vi "test-swerve-drive-kinematics-15.vi"() -> (3 "Test Passed":bool)   [LabVIEW 2019]
uses:
  <vilib>/Rock Robotics/WPI/ThirdParty/JAS_Junk/TrajLib/Conv_Deg_Radians.vi
  <vilib>/Rock Robotics/WPI/ThirdParty/JAS_Junk/TrajLib/Rotation2d_CreateAngle.vi
  <vilib>/Rock Robotics/WPI/ThirdParty/JAS_Junk/TrajLib/Trajectory_Library.lvlib
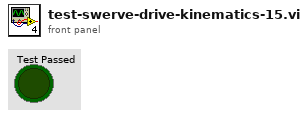
[diagram p1: front panel]
types:
  T1 = typedef "Trajectory_Library.lvlib/ROTATION2D.ctl" = cluster{"VALUE":dbl, "COS":dbl, "SIN":dbl}
  T2 = typedef "Trajectory_Library.lvlib/TRANSLATION2D.ctl" = cluster{"X":dbl, "Y":dbl}
  T3 = typedef "Trajectory_Library.lvlib/SWERVE_DRIVE_MODULE_POSITION.ctl" = cluster{"Distance":dbl, "Angle":T1}
  T4 = typedef "Trajectory_Library.lvlib/SWERVE_DRIVE_KINEMATICS.ctl" = cluster{"NumModules":i32, "InverseKinematics":T5, "ForwardKinematics":T5, "Modules":T2[], "PrevCoR":T2, "SavedModuleStates":T6[]}
  T5 = typedef "NI_Matrix.lvlib/RealMatrix.ctl" = dbl[][]
  T6 = typedef "Trajectory_Library.lvlib/SWERVE_DRIVE_MODULE_STATE.ctl" = cluster{"Speed":dbl, "Angle":T1}
  T7 = typedef "Trajectory_Library.lvlib/TWIST2D.ctl" = cluster{"dX":dbl, "dY":dbl, "dTHETA":dbl}
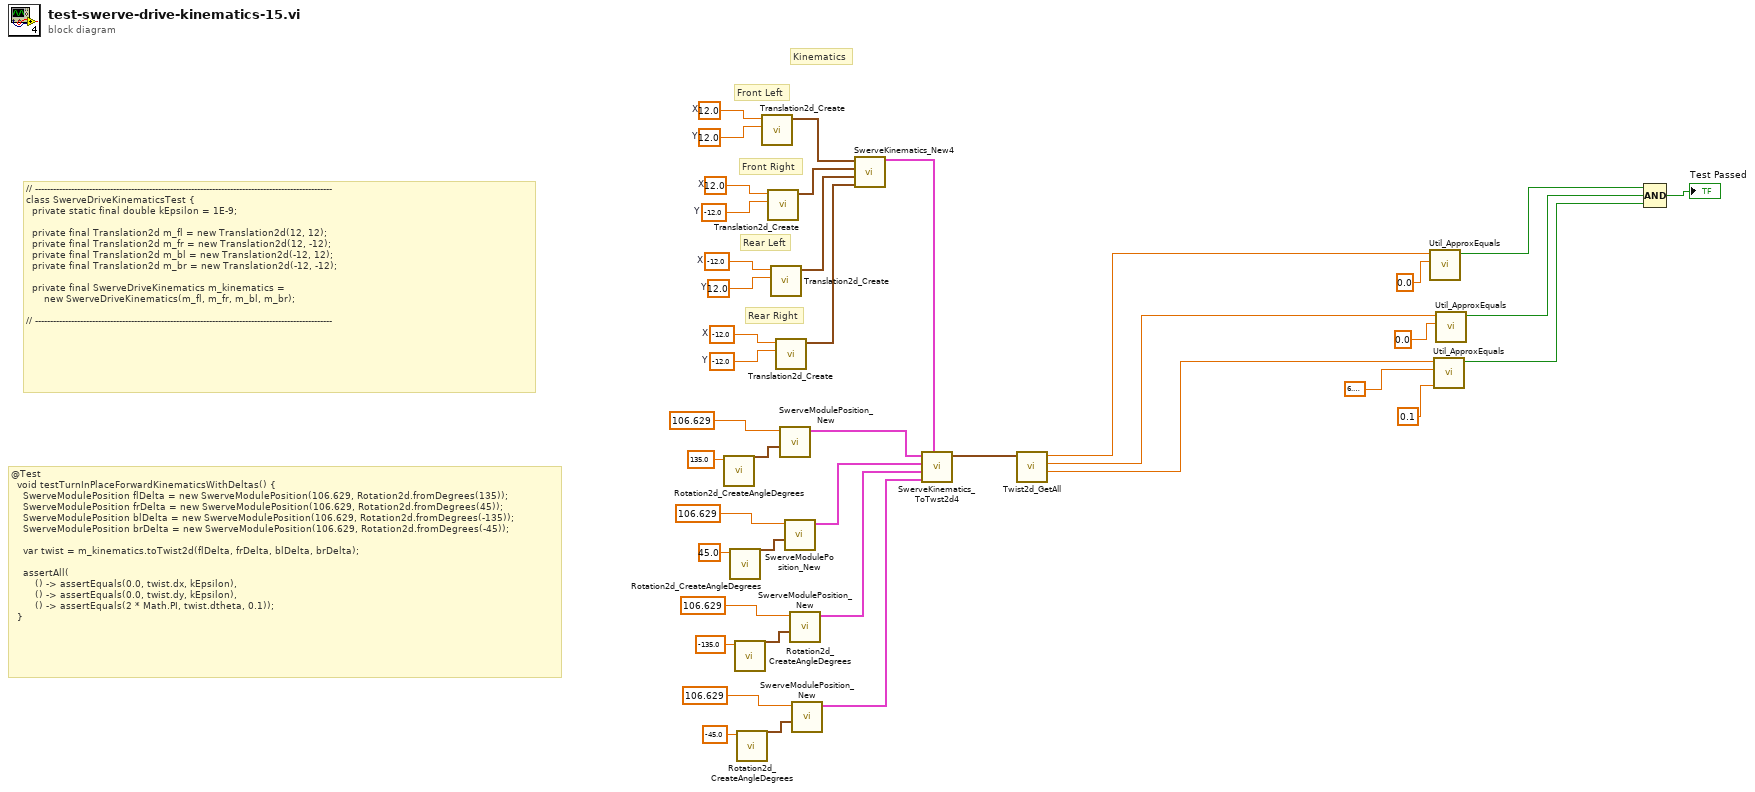
[diagram p0: block diagram]
diagram:
  w37 = -12.0  # X
  w36 = -12.0  # Y
  w35 = -12.0  # X
  w34 = 12.0  # Y
  w33 = 12.0  # X
  w32 = -12.0  # Y
  w31 = 12.0  # X
  w30 = 12.0  # Y
  # "@Test\n  void testTurnInPlaceForwardKinematicsWithDeltas() {\n    SwerveModulePosition flDelta = new SwerveModulePosition(106.629, Rotation2d.fromDegrees(135));\n    SwerveModulePosition frDelta = new SwerveModulePosition(106.629, Rotation2d.fromDegrees(45));\n    SwerveModulePosition blDelta = new SwerveModulePosition(106.629, Rotation2d.fromDegrees(-135));\n    SwerveModulePosition brDelta = new SwerveModulePosition(106.629, Rotation2d.fromDegrees(-45));\n\n    var twist = m_kinematics.toTwist2d(flDelta, frDelta, blDelta, brDelta);\n\n    assertAll(\n        () -> assertEquals(0.0, twist.dx, kEpsilon),\n        () -> assertEquals(0.0, twist.dy, kEpsilon),\n        () -> assertEquals(2 * Math.PI, twist.dtheta, 0.1));\n  }"
  # "Kinematics"
  # "Rear Right"
  # "Rear Left"
  # "Front Right"
  # "Front Left"
  # "// ---------------------------------------------------------------------------------------------------\nclass SwerveDriveKinematicsTest {\n  private static final double kEpsilon = 1E-9;\n\n  private final Translation2d m_fl = new Translation2d(12, 12);\n  private final Translation2d m_fr = new Translation2d(12, -12);\n  private final Translation2d m_bl = new Translation2d(-12, 12);\n  private final Translation2d m_br = new Translation2d(-12, -12);\n\n  private final SwerveDriveKinematics m_kinematics =\n      new SwerveDriveKinematics(m_fl, m_fr, m_bl, m_br);\n\n// ---------------------------------------------------------------------------------------------------"
  n1 = call <vilib>:"Rotation2d_CreateAngleDegrees.vi"("Angle_Degrees"=135.0) -> ("ROTATION"=w23:T1)  [unwired: 10 in]
  n2 = call <vilib>:"Rotation2d_CreateAngleDegrees.vi"("Angle_Degrees"=45.0) -> ("ROTATION"=w15:T1)  [unwired: 10 in]
  n3 = call <vilib>:"Rotation2d_CreateAngleDegrees.vi"("Angle_Degrees"=-135.0) -> ("ROTATION"=w12:T1)  [unwired: 10 in]
  n4 = call <vilib>:"Rotation2d_CreateAngleDegrees.vi"("Angle_Degrees"=-45.0) -> ("ROTATION"=w9:T1)  [unwired: 10 in]
  n5 = call <vilib>:"Translation2d_Create.vi"("Y"=w30, "X"=w31) -> ("TRANSLATION"=w38:T2)  [unwired: 9 in]
  n6 = call <vilib>:"Translation2d_Create.vi"("Y"=w32, "X"=w33) -> ("TRANSLATION"=w39:T2)  [unwired: 9 in]
  n7 = call <vilib>:"Translation2d_Create.vi"("Y"=w34, "X"=w35) -> ("TRANSLATION"=w40:T2)  [unwired: 9 in]
  n8 = call <vilib>:"Translation2d_Create.vi"("Y"=w36, "X"=w37) -> ("TRANSLATION"=w41:T2)  [unwired: 9 in]
  n9 = call <vilib>:"SwerveModulePosition_New.vi"("ROTATION"=w23, "Distance"=106.629 ("Speed")) -> ("SWERVE_DRIVE_MODULE_POSITION"=w6:T3)  [unwired: 9 in]
  n10 = call <vilib>:"SwerveModulePosition_New.vi"("ROTATION"=w15, "Distance"=106.629 ("Speed")) -> ("SWERVE_DRIVE_MODULE_POSITION"=w5:T3)  [unwired: 9 in]
  n11 = call <vilib>:"SwerveModulePosition_New.vi"("ROTATION"=w12, "Distance"=106.629 ("Speed")) -> ("SWERVE_DRIVE_MODULE_POSITION"=w4:T3)  [unwired: 9 in]
  n12 = call <vilib>:"SwerveModulePosition_New.vi"("ROTATION"=w9, "Distance"=106.629 ("Speed")) -> ("SWERVE_DRIVE_MODULE_POSITION"=w3:T3)  [unwired: 9 in]
  n13 = call <vilib>:"SwerveKinematics_New4.vi"("wheel 3"=w41, "wheel 2"=w40, "wheel 1"=w39, "wheel 0"=w38) -> ("SWERVE_DRIVE_KINEMATICS"=w20:T4)  [unwired: 7 in]
  n14 = call <vilib>:"SwerveKinematics_ToTwst2d4.vi"("in SWERVE_DRIVE_KINEMATICS"=w20, "Wheel Delta 3"=w3, "Wheel Delta 2"=w4, "Wheel Delta 1"=w5, "Wheel Delta 0"=w6) -> ("Twist2d"=w19:T7)  [unwired: 5 in, 1 out]
  n15 = call <vilib>:"Twist2d_GetAll.vi"("TWIST"=w19) -> ("dTHETA"=w16:dbl, "dY"=w17:dbl, "dX"=w18:dbl)  [unwired: 8 in]
  n16 = call <vilib>:"Util_ApproxEquals.vi"("Value 2"=0.0, "Value 1"=w18) -> ("ApproxEquals"=w27:bool)  [unwired: 9 in]
  n17 = call <vilib>:"Util_ApproxEquals.vi"("Tolerance"=0.1, "Value 2"=6.283185307179586, "Value 1"=w16) -> ("ApproxEquals"=w25:bool)  [unwired: 8 in]
  n18 = call <vilib>:"Util_ApproxEquals.vi"("Value 2"=0.0, "Value 1"=w17) -> ("ApproxEquals"=w26:bool)  [unwired: 9 in]
  n19 = Compound Arithmetic op=AND(w27, w26, w25) -> (→"Test Passed":bool)
